vi "浊度_所有参数读取.vi"(8 "error in (no error)":errorcluster caption="错误输入（无错误）", 11 "MB session in":refnum<class "MB_Master.lvclass">) -> (0 "error out":errorcluster caption="错误输出", 2 "输出值":T1 {"电极型号标志" items=["NULL", "pH", "Cond", "DO", "Turb"]; "电极状态标志" items=["OK"=0, "第一点校正通过"=1, "第二点校正通过"=2, "悬浮物两点校准第一点校正通过"=11, "悬浮物两点校准第二点校正通过"=12, "浊度三点校正第一点校正通过"=31, "浊度三点校正第二点校正通过"=32, "浊度三点校正第三点校正通过"=33]}, 3 "MB session out":refnum<class "MB_Master.lvclass">)   [LabVIEW 2016, in "斯坦道多参数.lvlib"]
uses:
  <vilib>/Plasmionique/MB Master/MB_Master/MB_Master.lvclass
  <vilib>/Plasmionique/MB Master/MB Master.lvlib
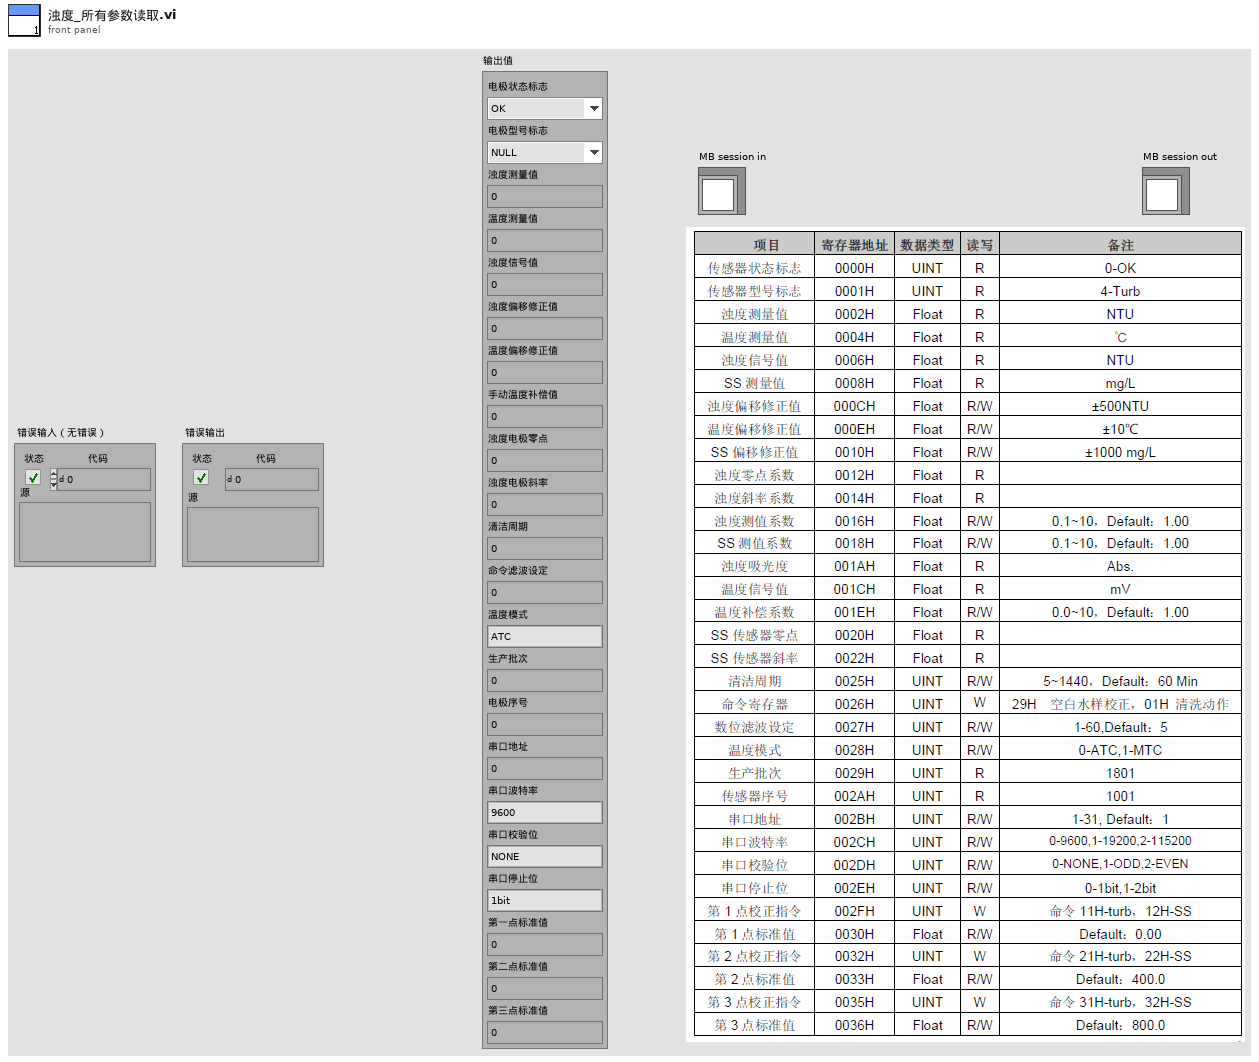
[diagram p1: front panel]
types:
  T1 = cluster{"电极状态标志":u16, "电极型号标志":u16, "浊度测量值":sgl, "温度测量值":sgl, "浊度信号值":sgl, "浊度偏移修正值":sgl, "温度偏移修正值":sgl, "手动温度补偿值":sgl, "浊度电极零点":sgl, "浊度电极斜率":sgl, "清洁周期":u16, "命令滤波设定":u16, "温度模式":enum16{"ATC", "MTC"}, "生产批次":u16, "电极序号":u16, "串口地址":u16, "串口波特率":enum16{"9600", "19200", "115200"}, "串口校验位":enum16{"NONE", "ODD", "EVEN"}, "串口停止位":enum16{"1bit", "2bit"}, "第一点标准值":sgl, "第二点标准值":sgl, "第三点标准值":sgl}
  T2 = cluster{u16, u16, "数值":sgl, "数值":sgl, "数值":sgl, "数值":sgl, "数值":sgl, "数值":sgl, "数值":sgl, "数值":sgl, u16, u16, u16, u16, u16, u16, u16, u16, u16, "数值":sgl, "数值":sgl, "数值":sgl}
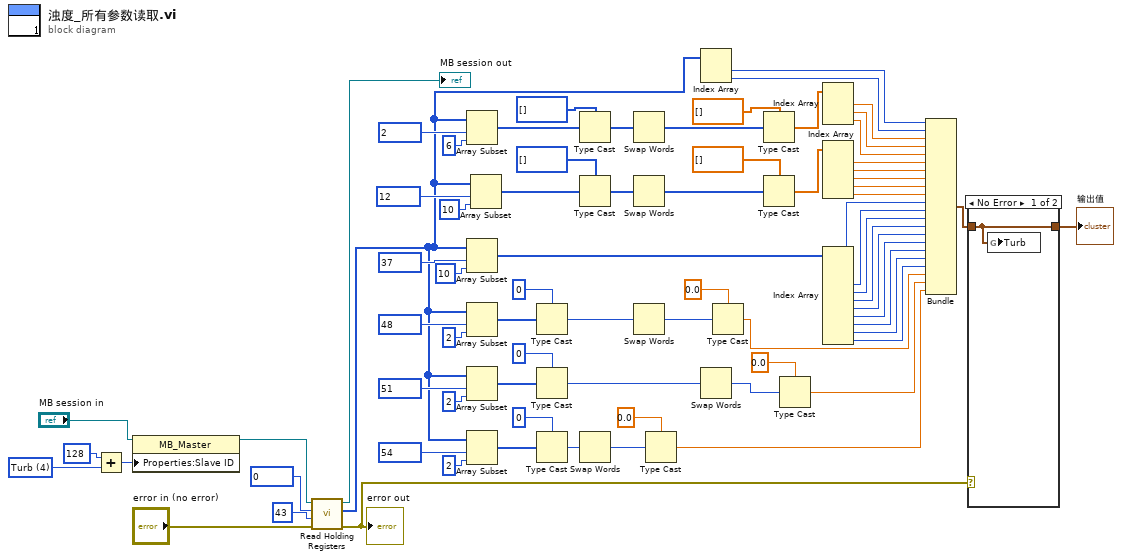
[diagram p0: block diagram]
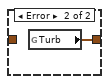
[diagram p2: hidden frame]
diagram:
  w75 = u16 4 items=["NULL", "pH", "Cond", "DO", "Turb"] ("数值")
  n1 = Add(x=u16 128, y=w75) -> (x+y=w74:u16)
  n2 = property class="MB_Master"(reference="MB session in", "Properties:Slave ID"=w74) -> (reference out=w17:refnum<class "MB_Master.lvclass">)  [unwired: 1 in, 1 out]
  n3 = call <vilib>:"Read Holding Registers.vi"("error in (no error)"="error in (no error)", "quantity"=u16 43, "starting address"=u16 0, "MB session in"=w17) -> ("error out"=w16:errorcluster, "Registers"=w2:u16[], "MB session out"=→"MB session out":refnum<class "MB_Master.lvclass">)  [unwired: 5 in]
  "error out" <- w16
  n4 = Array Subset(array=w2, index=u16 2 ("starting address"), length=6 ("长度")) -> (w63:u16[])
  n5 = Array Subset(array=w2, index=u16 37 ("starting address"), length=10 ("长度")) -> (w43:u16[])
  n6 = Array Subset(array=w2, index=u16 48 ("starting address"), length=2 ("长度")) -> (w26:u16[])
  n7 = Array Subset(array=w2, index=u16 51 ("starting address"), length=2 ("长度")) -> (w21:u16[])
  n8 = Array Subset(array=w2, index=u16 54 ("starting address"), length=2 ("长度")) -> (w14:u16[])
  n9 = Array Subset(array=w2, index=u16 12 ("starting address"), length=10 ("长度")) -> (w54:u16[])
  n10 = Type Cast(type=u32 0 ("数值"), x=w26) -> (*(type *) &x=w29:u32)
  n11 = Type Cast(type=u32 0 ("数值"), x=w21) -> (*(type *) &x=w23:u32)
  n12 = Type Cast(type=u32 0 ("数值"), x=w14) -> (*(type *) &x=w12:u32)
  n13 = Type Cast(type=u32[] [] ("数组 2"), x=w63) -> (*(type *) &x=w65:u32[])
  n14 = Type Cast(type=u32[] [] ("数组 2"), x=w54) -> (*(type *) &x=w57:u32[])
  n15 = Swap Words(1:w12) -> (0:w13:u32)
  n16 = Swap Words(1:w65) -> (0:w67:u32[])
  n17 = Swap Words(1:w57) -> (0:w58:u32[])
  n18 = Swap Words(1:w29) -> (0:w30:u32)
  n19 = Type Cast(type=sgl 0.0 ("数值"), x=w13) -> (*(type *) &x=w7:sgl)
  n20 = Index Array(array=w2) -> (element #1=w70:u16, element #2=w69:u16)  [unwired: 2 in]
  n21 = Swap Words(1:w23) -> (0:w22:u32)
  n22 = Type Cast(type=sgl 0.0 ("数值"), x=w30) -> (*(type *) &x=w20:sgl)
  n23 = Type Cast(type=sgl[] [] ("数组 2"), x=w67) -> (*(type *) &x=w62:sgl[])
  n24 = Type Cast(type=sgl[] [] ("数组 2"), x=w58) -> (*(type *) &x=w53:sgl[])
  n25 = Type Cast(type=sgl 0.0 ("数值"), x=w22) -> (*(type *) &x=w19:sgl)
  n26 = Index Array(array=w62) -> (element #1=w4:sgl, element #2=w61:sgl, element #3=w60:sgl)  [unwired: 3 in]
  n27 = Index Array(array=w53) -> (element #1=w52:sgl, element #2=w51:sgl, element #3=w50:sgl, element #4=w49:sgl, element #5=w48:sgl)  [unwired: 5 in]
  n28 = Index Array(array=w43) -> (element #1=w1:u16, element #3=w42:u16, element #4=w41:u16, element #5=w40:u16, element #6=w39:u16, element #7=w38:u16, element #8=w37:u16, element #9=w36:u16, element #10=w35:u16)  [unwired: 10 in, 1 out]
  n29 = Bundle(w70, w69, "数值"=w4, "数值"=w61, "数值"=w60, "数值"=w52, "数值"=w51, "数值"=w50, "数值"=w49, "数值"=w48, w1, w42, w41, w40, w39, w38, w37, w36, w35, "数值"=w20, "数值"=w19, "数值"=w7) -> (w15:T2)  [unwired: 1 in]
  n30 = case shown="No Error" w16 {
    tunnel: w15 -> [w76 _]
    tunnel: [w76 w77] -> w3
    frame No Error {
      n31 = global write "国弘过程全局变量.vi" "Turb"(w76) -> ()
    }
    frame Error {
      n32 = global read "国弘过程全局变量.vi" "Turb"() -> (w77:T1)
    }
  }
  "输出值" <- w3
